vi "GPIB_autodetect.vi"(8 "error in (no error)":errorcluster, 9 "Verify GPIB address":bool, 10 "Instrument GPIB address in":string, 11 "InstrControl in":refnum<class "InstrControl.lvclass">) -> (0 "error out":errorcluster, 2 "Instrument GPIB address":string, 3 "InstrControl out":refnum<class "InstrControl.lvclass">)   [LabVIEW 2013, in "InstrControl.lvclass"]
uses:
  InstrControl.lvclass
panel:
  out "instrument responses":string[](array[string])
  out "GPIB addresses found":string[](array[string])
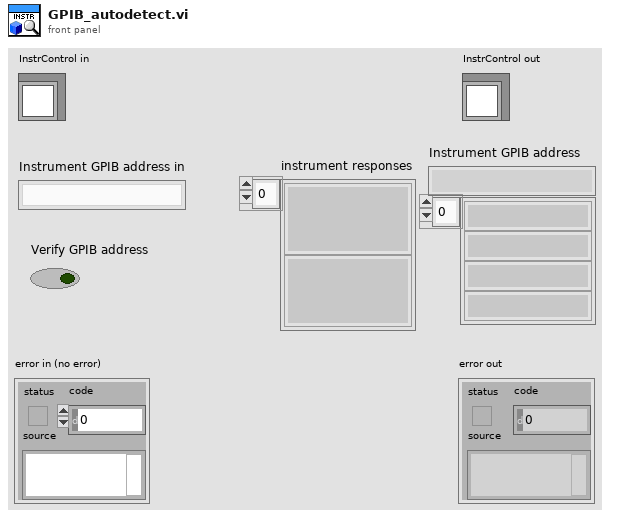
[diagram p1: front panel]
types:
  T1 = cluster{"error":bool, "code":i32, "source":string}
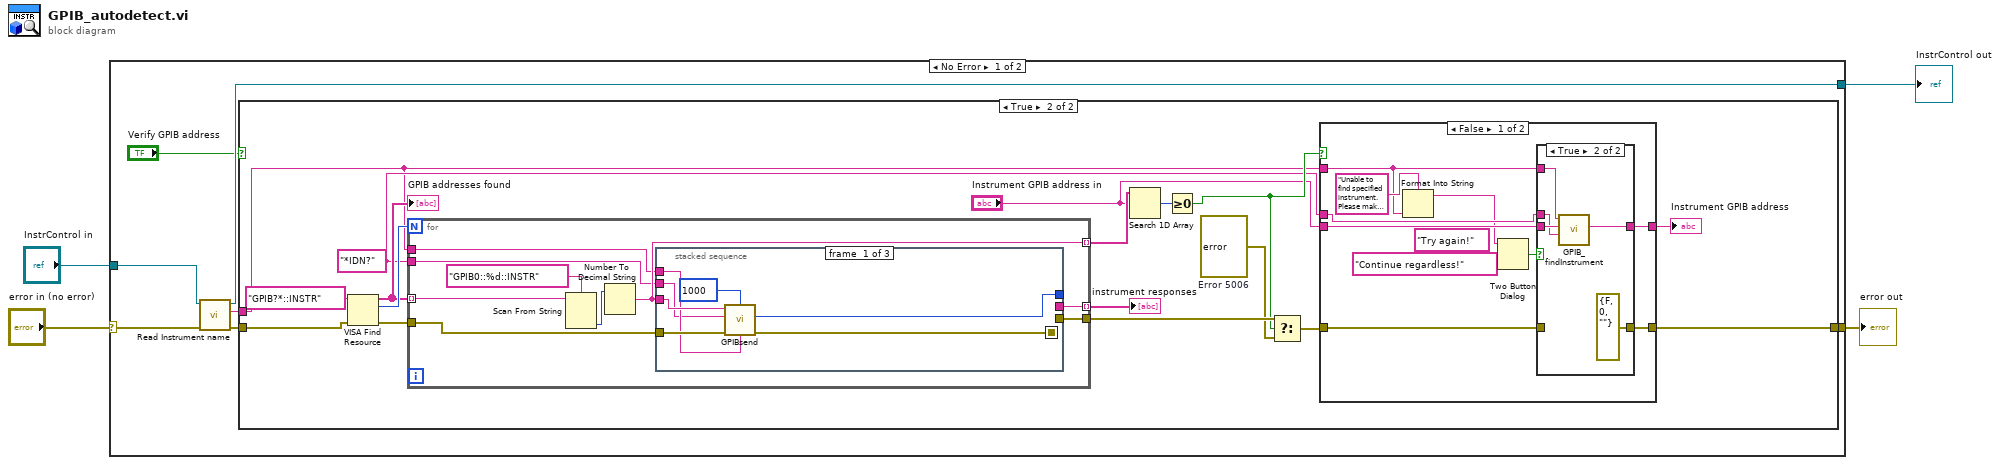
[diagram p0: block diagram]
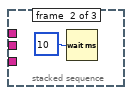
[diagram p5: hidden frame]
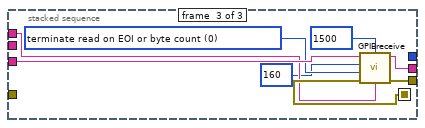
[diagram p6: hidden frame]
diagram:
  n1 = case shown="No Error" "error in (no error)" {
    selector: "error in (no error)" -> [w10 w76]
    tunnel: [w7 w76] -> w3
    tunnel: [w9 w75] -> w1
    tunnel: "InstrControl in" -> [w11 w75]
    frame No Error {
      n2 = call-dynamic "Read Instrument name.vi"("error in (no error)"=w10, "InstControl in"=w11) -> ("error out"=w8:errorcluster, "Instrument name"=w6:string, "InstControl out"=w9:refnum<class "InstrControl.lvclass">)  [unwired: 7 in]
      n3 = case shown="True" "Verify GPIB address" {
        tunnel: w8 -> [w12 w23]
        tunnel: [w12 w15] -> w7
        tunnel: w6 -> [_ w13]
        frame False {
        }
        frame True {
          w14 = "*IDN?" ("regular expression")
          w28 = errorcluster {"status"=FALSE, "code"=5005, "source"="Unable to find specified instrument.  Please make sure the it is connected to your system and switched on."}  # Error 5006
          n4 = VISA Find Resource(8:w23, 11:"GPIB?*::INSTR" ("expression (\"\")")) -> (0:w27:errorcluster, 2:w26:u32, 3:w25:string[])  [unwired: 1 in]
          "GPIB addresses found" <- w25
          n5 = for {
            N: w26 -> [_]
            tunnel: w25 -> [w56] mode=indexing
            tunnel: w27 -> [w58]
            tunnel: [w57] -> w29
            tunnel: [w52] -> w20 mode=indexing
            tunnel: w13 -> [w51]
            tunnel: [w53] -> w24 mode=indexing
            tunnel: w14 -> [w50]
            n6 = Scan From String(format string="GPIB0::%d::INSTR" ("expression (\"\")"), input string=w56) -> (output 1=w54:i32)  [unwired: 3 in, 3 out]
            n7 = Number To Decimal String(number=w54) -> (decimal integer string=w52:string)  [unwired: 1 in]
            n8 = stacked-sequence {
              seq-local: [w63 _ _] -> [_ _ w73]
              tunnel: w52 -> [w65 _ w72]
              tunnel: w58 -> [w64 _ _]
              tunnel: [_ _ w74] -> w57
              tunnel: [_ _ w69] -> w53
              tunnel: w51 -> [w61 _ w70]
              tunnel: w50 -> [w60 _ _]
              tunnel: [w59 _ _] -> _
              frame #0 {
                n9 = call "GPIBsend.vi"("timeout ms"=u32 1000, "address string"=w65, "write buffer"=w60, "source"=w61, "error in"=w64) -> ("byte count"=w59:i32, "error out"=w63:errorcluster)  [unwired: 2 in, 1 out]
              }
              frame #1 {
                n10 = Wait (ms)(milliseconds to wait=10) -> ()  [unwired: 1 out]
              }
              frame #2 {
                w68 = 0 items=["terminate read on EOI or byte count", "terminate read on EOI, byte count, or CR", "terminate read on EOI, byte count, or LF"] ("read mode")
                n11 = call "GPIBreceive.vi"("timeout ms"=u32 1500, "address string"=w72, "byte count"=160, "source"=w70, "read mode"=w68, "error in"=w73) -> ("read buffer"=w69:string, "error out"=w74:T1)  [unwired: 1 in, 1 out]
              }
            }
          }
          "instrument responses" <- w24
          n12 = Search 1D Array(1D array=w20, element="Instrument GPIB address in") -> (index of element=w19:i32)  [unwired: 1 in]
          n13 = Greater Or Equal To 0?(x=w19) -> (x >= 0?=w18:bool)
          n14 = Select(t=w29, s=w18, f=w28) -> (s? t:f=w16:errorcluster)
          n15 = case shown="False" w18 {
            tunnel: "Instrument GPIB address in" -> [w37 w49]
            tunnel: [w36 w49] -> w21
            tunnel: w16 -> [w35 w48]
            tunnel: [w34 w48] -> w15
            tunnel: w14 -> [w33 _]
            tunnel: w13 -> [w31 _]
            frame False {
              n16 = Format Into String(format string="Unable to find specified instrument.  Please make sure the it is connected to your system and switched on.\n\n%s" ("source"), w31) -> (resulting string=w30:string)  [unwired: 2 in, 1 out]
              n17 = Two Button Dialog(message=w30, 1:"Continue regardless!", 2:"Try again!") -> (T button?=w38:bool)
              n18 = case shown="True" w38 {
                tunnel: w37 -> [w42 w47]
                tunnel: [w42 w46] -> w36
                tunnel: w35 -> [w41 _]
                tunnel: [w41 errorcluster {"status"=FALSE, "code"=0, "source"=""} ("error constant")] -> w34
                tunnel: w33 -> [_ w44]
                tunnel: w31 -> [_ w43]
                frame False {
                }
                frame True {
                  n19 = call "GPIB_findInstrument.vi"("ID command"=w44, "revised GPIB address"=w47, "Instrument name IN"=w43) -> ("revised GPIB address OUT"=w46:string)  [unwired: 8 in]
                }
              }
            }
            frame True {
            }
          }
          "Instrument GPIB address" <- w21
        }
      }
    }
    frame Error {
    }
  }
  "error out" <- w3
  "InstrControl out" <- w1
